vi "Write Chnl Obj.vi"(8 "error in (no error)":errorcluster, 10 "BME_DG_Chnl":refnum<class "BME_DG_Chnl.lvclass">, 11 "BME_DG_Base in":refnum<class "BME_DG_Base.lvclass">) -> (0 "error out":errorcluster, 3 "BME_DG_Base out":refnum<class "BME_DG_Base.lvclass">)   [LabVIEW 2009, in "POLARIS BME DG.lvlib" / "BME_DG_Base.lvclass"]
uses:
  BME_DG_Base.lvclass
  BME_DG_Chnl/BME_DG_Chnl.lvclass
  BME_DG_Base.lvclass/BME_DG_Base.ctl
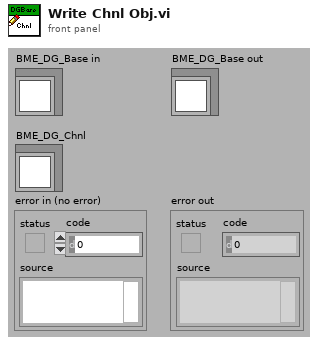
[diagram p1: front panel]
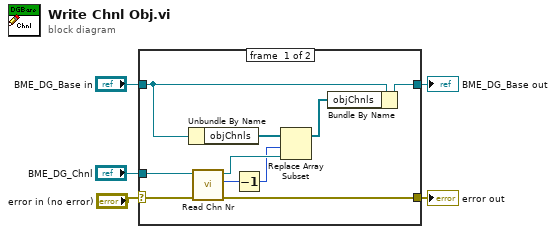
[diagram p0: block diagram]
diagram:
  n1 = case shown="No Error" "error in (no error)" {
    selector: "error in (no error)" -> [w10 w17]
    tunnel: [w9 w17] -> w4
    tunnel: [w8 w16] -> w2
    tunnel: "BME_DG_Base in" -> [w15 w16]
    tunnel: "BME_DG_Chnl" -> [w12 _]
    frame #0 {
      n2 = Unbundle By Name(w15) -> ("objChnls"=w14:refnum<class "BME_DG_Chnl.lvclass">[])
      n3 = call-dynamic "Read Chn Nr.vi"("error in (no error)"=w10, "BME_DG_Chnl in"=w12) -> ("error out"=w9:errorcluster, "Chn Nr"=w13:i32, "BME_DG_Chnl out"=w11:refnum<class "BME_DG_Chnl.lvclass">)  [unwired: 7 in]
      n4 = Decrement(x=w13) -> (x-1=w6:i32)
      n5 = Replace Array Subset(array=w14, new element=w11, index=w6) -> (w7:refnum<class "BME_DG_Chnl.lvclass">[])
      n6 = Bundle By Name(cluster=w15, "objChnls"=w7) -> (w8:refnum<class "BME_DG_Base.lvclass">)
    }
    frame #1 {
    }
  }
  "error out" <- w4
  "BME_DG_Base out" <- w2
